vi "Get_Labels_from_subFolders_Names.vi"(11 "All Files in Dir":path[](array[path])) -> (3 "Labels":string[](array[string]))   [LabVIEW 2020]
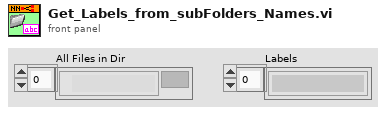
[diagram p1: front panel]
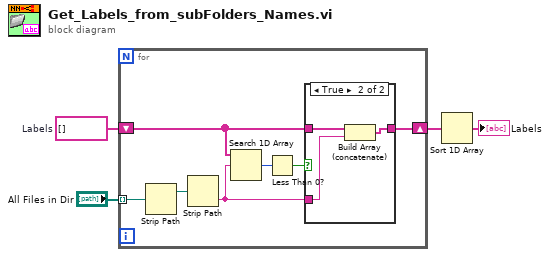
[diagram p0: block diagram]
diagram:
  w3 = string[] []  # Labels
  n1 = for {
    tunnel: "All Files in Dir" -> [w10] mode=indexing
    shift-right: [w5] -> w4
    shift-left: w3 -> [w7]
    n2 = Strip Path(path=w10) -> (stripped path=w11:path)  [unwired: 1 out]
    n3 = Strip Path(path=w11) -> (name=w6:string)  [unwired: 1 out]
    n4 = Search 1D Array(1D array=w7, element=w6) -> (index of element=w9:i32)  [unwired: 1 in]
    n5 = Less Than 0?(x=w9) -> (x < 0?=w8:bool)
    n6 = case shown="True" w8 {
      tunnel: [w12 w15] -> w5
      tunnel: w7 -> [w12 w14]
      tunnel: w6 -> [_ w13]
      frame False {
      }
      frame True {
        n7 = Build Array (concatenate)(w14, w13) -> (w15:string[])
      }
    }
  }
  n8 = Sort 1D Array(array=w4) -> (sorted array=→"Labels":string[])
